vi "Vessel Visualization.vi"() -> ()   [LabVIEW 2014]
uses:
  <vilib>/picture/3D Picture Control/NI_3D Picture Control.lvlib
panel:
  in  "Scale DOF":dbl[](array[numeric])
  in  "Scale Thruster":dbl[](array[numeric])
  in  "Thruster Vector":bool
  out "3D Picture":refnum<vi>(3d-picture)
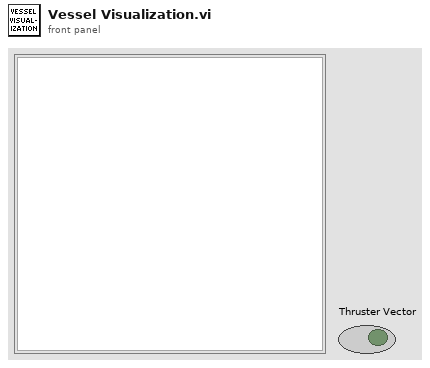
[diagram p1: front panel]
types:
  T1 = cluster{"Numeric":dbl, "Numeric":dbl, "Numeric":dbl}
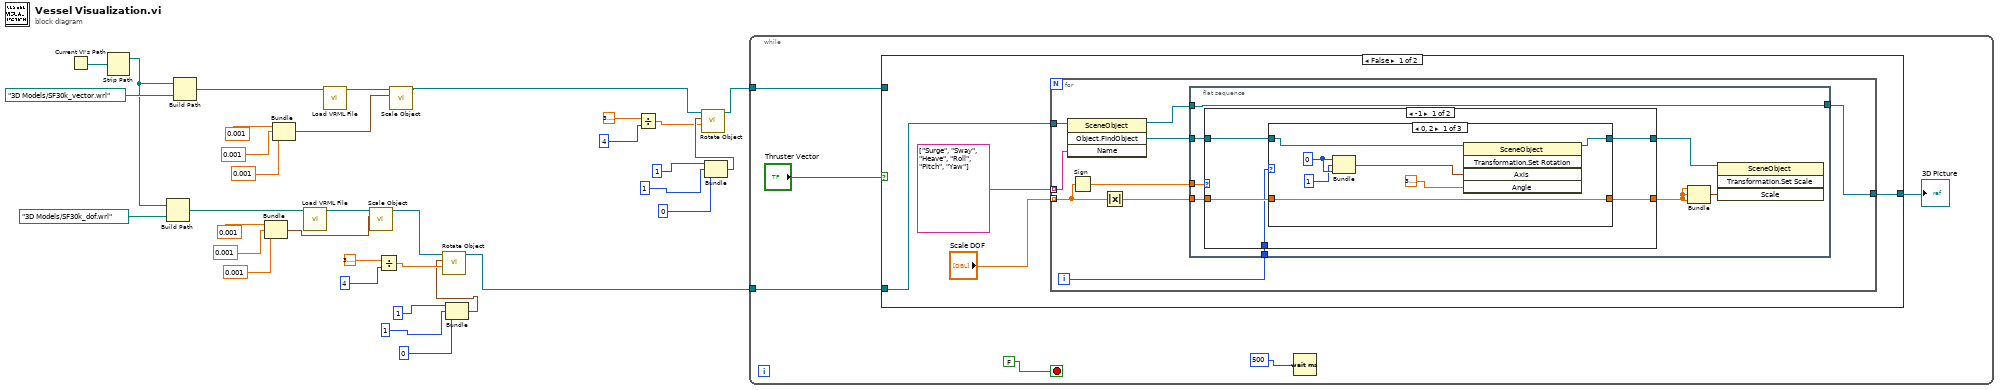
[diagram p0: block diagram]
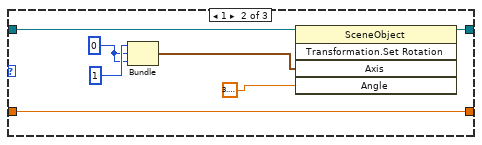
[diagram p2: hidden frame]
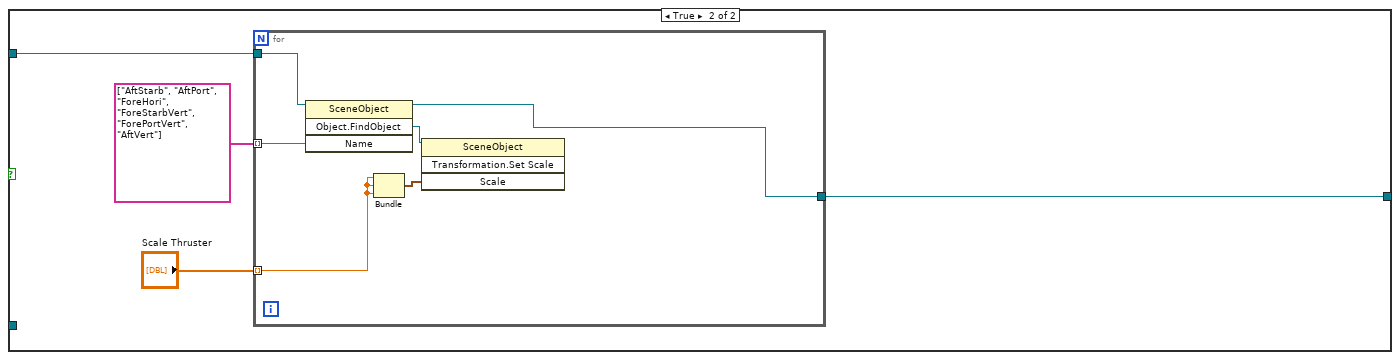
[diagram p5: hidden frame]
diagram:
  n1 = Current VI's Path() -> (path=w2:path)
  n2 = Strip Path(path=w2) -> (stripped path=w1:path)  [unwired: 1 out]
  n3 = Build Path(base path=w1, name or relative path=path "3D Models/SF30k_dof.wrl") -> (appended path=w3:path)
  n4 = Build Path(base path=w1, name or relative path=path "3D Models/SF30k_vector.wrl") -> (appended path=w5:path)
  n5 = Bundle(0.001, 0.001, 0.001) -> (w29:cluster{dbl, dbl, dbl})  [unwired: 1 in]
  n6 = Bundle(0.001, 0.001, 0.001) -> (w33:cluster{dbl, dbl, dbl})  [unwired: 1 in]
  n7 = call <vilib>:"Load VRML File.vi"("Path"=w3) -> ("Scene:Read Scene File"=w25:refnum<vi>)  [unwired: 9 in, 1 out]
  n8 = call <vilib>:"Load VRML File.vi"("Path"=w5) -> ("Scene:Read Scene File"=w34:refnum<vi>)  [unwired: 9 in, 1 out]
  n9 = call <vilib>:"Scale Object.vi"("Scale"=w29, "Scene.Object In"=w25) -> ("Scene.Object Out"=w9:refnum<vi>)  [unwired: 8 in, 1 out]
  n10 = Divide(x=3.141592653589793, y=4) -> (x/y=w10:dbl)
  n11 = call <vilib>:"Scale Object.vi"("Scale"=w33, "Scene.Object In"=w34) -> ("Scene.Object Out"=w23:refnum<vi>)  [unwired: 8 in, 1 out]
  n12 = Bundle(1, 1, 0) -> (w8:cluster{i32, i32, i32})  [unwired: 1 in]
  n13 = call <vilib>:"Rotate Object.vi"("Angle"=w10, "Axis"=w8, "Scene.Object In"=w9) -> ("Scene.Object Out"=w7:refnum<vi>)  [unwired: 7 in, 1 out]
  n14 = Divide(x=3.141592653589793, y=4) -> (x/y=w16:dbl)
  n15 = Bundle(1, 1, 0) -> (w19:cluster{i32, i32, i32})  [unwired: 1 in]
  n16 = call <vilib>:"Rotate Object.vi"("Angle"=w16, "Axis"=w19, "Scene.Object In"=w23) -> ("Scene.Object Out"=w22:refnum<vi>)  [unwired: 7 in, 1 out]
  n17 = while {
    tunnel: w22 -> [w39]
    tunnel: w7 -> [w38]
    stop <- FALSE stop-if-true
    n18 = case shown="False" "Thruster Vector" {
      tunnel: [w42 w88] -> w37
      tunnel: w39 -> [_ w87]
      tunnel: w38 -> [w43 _]
      frame False {
        n19 = for {
          tunnel: string[] ["Surge", "Sway", "Heave", "Roll", "Pitch", "Yaw"] -> [w51] mode=indexing
          tunnel: w43 -> [w52]
          tunnel: [w45] -> w42
          tunnel: "Scale DOF" -> [w50] mode=indexing
          i -> [w48]
          n20 = invoke class="SceneObject" method="Object.FindObject"(reference=w52, "Name"=w51) -> (reference out=w46:refnum<vi>, "FindObject"=w47:refnum<vi>)  [unwired: 2 in, 2 out]
          n21 = Sign(1:w50) -> (0:w53:dbl)
          n22 = Absolute Value(x=w50) -> (abs(x)=w49:dbl)
          n23 = flat-sequence {
            tunnel: w53 -> [w61]
            tunnel: w49 -> [w58]
            tunnel: w48 -> [w57]
            tunnel: w47 -> [w56]
            tunnel: w46 -> [w54]
            tunnel: [w54] -> w45
            frame #0 {
              n24 = case shown="-1" w61 {
                tunnel: w58 -> [w66 w84]
                tunnel: [w65 w84] -> w59
                tunnel: w56 -> [w63 w83]
                tunnel: [w62 w83] -> w55
                tunnel: w57 -> [w64 _]
                frame -1 {
                  n25 = case shown="0, 2" w64 {
                    tunnel: w66 -> [w72 w80 w82]
                    tunnel: [w72 w80 w82] -> w65
                    tunnel: w63 -> [w73 w79 w81]
                    tunnel: [w67 w74 w81] -> w62
                    frame 0, 2 {
                      w70 = 0
                      n26 = Bundle(w70, 1, w70) -> (w71:cluster{i32, i32, i32})  [unwired: 1 in]
                      n27 = invoke class="SceneObject" method="Transformation.Set Rotation"(reference=w73, "Axis"=w71, "Angle"=3.141592653589793) -> (reference out=w67:refnum<vi>)  [unwired: 2 in, 4 out]
                    }
                    frame 1 {
                      w75 = 0
                      n28 = Bundle(1, w75, w75) -> (w78:cluster{i32, i32, i32})  [unwired: 1 in]
                      n29 = invoke class="SceneObject" method="Transformation.Set Rotation"(reference=w79, "Axis"=w78, "Angle"=3.141592653589793) -> (reference out=w74:refnum<vi>)  [unwired: 2 in, 4 out]
                    }
                    frame 3..5, Default {
                    }
                  }
                }
                frame 0, 1, Default {
                }
              }
              n30 = Bundle(w59, w59, w59) -> (w60:cluster{dbl, dbl, dbl})  [unwired: 1 in]
              n31 = invoke class="SceneObject" method="Transformation.Set Scale"(reference=w55, "Scale"=w60) -> ()  [unwired: 2 in, 4 out]
            }
          }
        }
      }
      frame True {
        n32 = for {
          tunnel: [w90] -> w88
          tunnel: w87 -> [w92]
          tunnel: string[] ["AftStarb", "AftPort", "ForeHori", "ForeStarbVert", "ForePortVert", "AftVert"] -> [w91] mode=indexing
          tunnel: "Scale Thruster" -> [w89] mode=indexing
          n33 = invoke class="SceneObject" method="Object.FindObject"(reference=w92, "Name"=w91) -> (reference out=w90:refnum<vi>, "FindObject"=w93:refnum<vi>)  [unwired: 2 in, 2 out]
          n34 = Bundle("Numeric"=w89, "Numeric"=w89, "Numeric"=w89) -> (w94:T1)  [unwired: 1 in]
          n35 = invoke class="SceneObject" method="Transformation.Set Scale"(reference=w93, "Scale"=w94) -> ()  [unwired: 2 in, 4 out]
        }
      }
    }
    "3D Picture" <- w37
    n36 = Wait (ms)(milliseconds to wait=500) -> ()  [unwired: 1 out]
  }
